vi "nearCamSetSoftwareTrigger.vi"(3 "错误输入（无错误）":errorcluster, 5 "IMAQdx Session":T1) -> (0 "错误输出":errorcluster, 2 "IMAQdx Session Out":T1)   [LabVIEW 2018]
uses:
  <vilib>/userdefined/High Color/IMAQdx.ctl
  <resource>/objmgr/imaqdx.rc
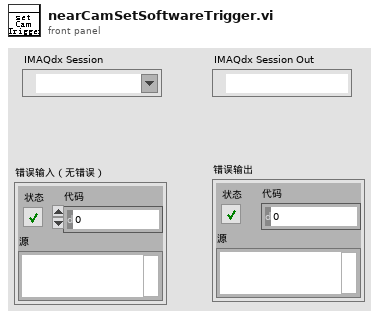
[diagram p1: front panel]
types:
  T1 = typedef "IMAQdx.ctl" = refnum<k21>
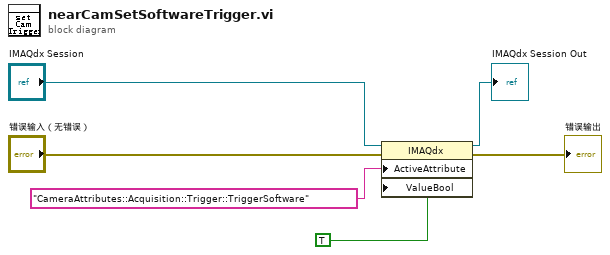
[diagram p0: block diagram]
diagram:
  n1 = property class="IMAQdx"(reference="IMAQdx Session", error in="错误输入（无错误）", "ActiveAttribute"="CameraAttributes::Acquisition::Trigger::TriggerSoftware", "ValueBool"=TRUE) -> (reference out=→"IMAQdx Session Out":T1, error out=→"错误输出":errorcluster)
